vi "To JSON.vi"(8 "error in":errorcluster, 11 "Theme Config in":refnum<class "Theme Config.lvclass">) -> (0 "error out":errorcluster, 2 "JSON":string, 3 "Theme Config out":refnum<class "Theme Config.lvclass">)   [LabVIEW 2021, in "Theme Config.lvclass"]
doc: "Convert the class data into a cluster that can be easily flattened to json using the jsontext toolkit.\n\n<b>Code Developed By:</b> +\nDaniel Coons +\nTechnology Service Corporation +\nwww.tsc.com/atcs"
uses:
  Theme Config.lvclass
  Theme Config.lvclass/Theme Config.ctl
  <vilib>/JDP Science/JSONtext/JSONtext.lvlib
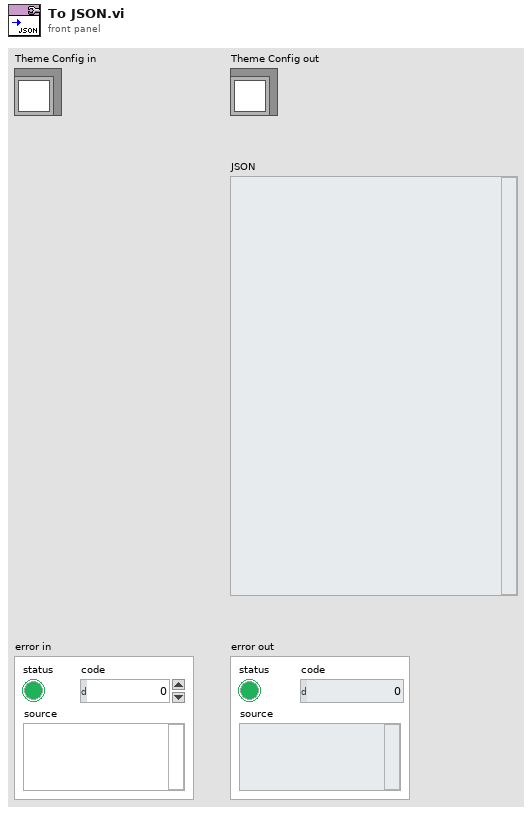
[diagram p1: front panel]
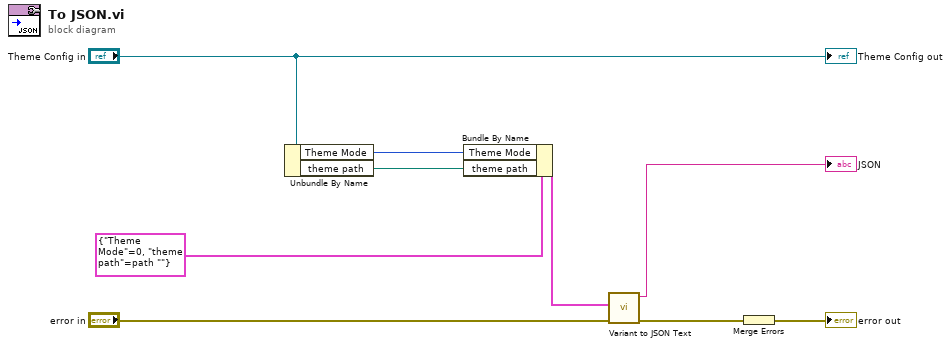
[diagram p0: block diagram]
diagram:
  n1 = Unbundle By Name("Theme Config in") -> ("Theme Mode"=w4:u16, "theme path"=w3:path)
  n2 = Bundle By Name(cluster=cluster{"Theme Mode":u16, "theme path":path} {"Theme Mode"=0, "theme path"=path ""} ("Cluster of class private data"), "Theme Mode"=w4, "theme path"=w3) -> (w1:cluster{"Theme Mode":u16, "theme path":path})
  n3 = call <vilib>:"Variant to JSON Text.vi"("error in (no error)"="error in", "Variant"=w1) -> ("error out"=w7:errorcluster, "<JSON>"=→"JSON":string)  [unwired: 7 in, 1 out]
  n4 = Merge Errors(w7) -> (→"error out":errorcluster)
  "Theme Config out" <- "Theme Config in"
